vi "Element Analog Table.vi"(8 "error in (no error)":errorcluster) -> (0 "error out":errorcluster, 3 "element":i64)   [LabVIEW 2020, in "Settings.lvlib"]
uses:
  Settings.lvlib
  <vilib>/drjdpowell/SQLite Library/SQL Connection/Open (path).vi
  <vilib>/drjdpowell/SQLite Library/SQL Connection/Open (string).vi
  <vilib>/AdvancedString/Path To Command Line String.vi
  <vilib>/drjdpowell/SQLite Library/SQL Connection/Execute SQL (1D Integer results).vi
  <vilib>/drjdpowell/SQLite Library/SQL Connection/Connection.lvclass
  <vilib>/drjdpowell/SQLite Library/SQLite.lvlib
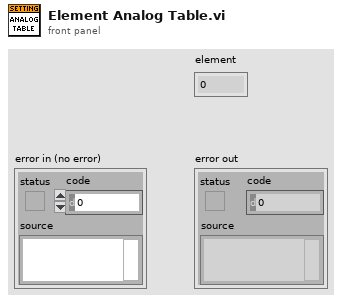
[diagram p1: front panel]
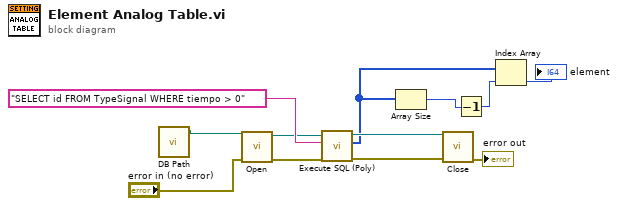
[diagram p0: block diagram]
diagram:
  n1 = call "DB Path.vi"() -> ("DB path"=w12:path)  [unwired: 11 in]
  n2 = call-poly <vilib>:"Open.vi"("error in (no error)"="error in (no error)", "db file"=w12) -> ("error out"=w6:errorcluster, "SQLite Connection"=w7:refnum<class "Connection.lvclass">)  [unwired: 8 in]
  n3 = call-poly <vilib>:"Execute SQL (Poly).vi"("error in (no error)"=w6, "SQL"="SELECT id FROM TypeSignal WHERE tiempo > 0", "SQLite Connection in"=w7) -> ("error out"=w9:errorcluster, "Result Set"=w2:i64[], "SQLite Connection"=w8:refnum<class "Connection.lvclass">)  [unwired: 5 in, 1 out]
  n4 = Array Size(array=w2) -> (size(s)=w4:i32)
  n5 = call-dynamic "Close.vi"("error in (no error)"=w9, "SQLite Connection in"=w8) -> ("error out"=→"error out":errorcluster)  [unwired: 9 in]
  n6 = Decrement(x=w4) -> (x-1=w3:i32)
  n7 = Index Array(array=w2, index=w3) -> (element=→"element":i64)
